vi "Construct.vi"(8 "error in (no error)":errorcluster, 11 "gRPCid":T1) -> (0 "error out":errorcluster, 3 "GRPCMessage out":refnum<class "GRPCMessage.lvclass">)   [LabVIEW 2019, in "MicronGRPCServer.lvlib" / "GRPCMessage.lvclass"]
uses:
  GRPCMessage.lvclass
  <vilib>/gRPC/LabVIEW gRPC Library/Shared/grpcId.ctl
  GRPCMessage.lvclass/GRPCMessage.ctl
  Service/Generated/MicronGRPCGeneratedServer/RPC Service/MicronGRPC/MicronGRPC.lvclass
  <vilib>/gRPC/LabVIEW gRPC Library/grpc-lvsupport-release.lvlib
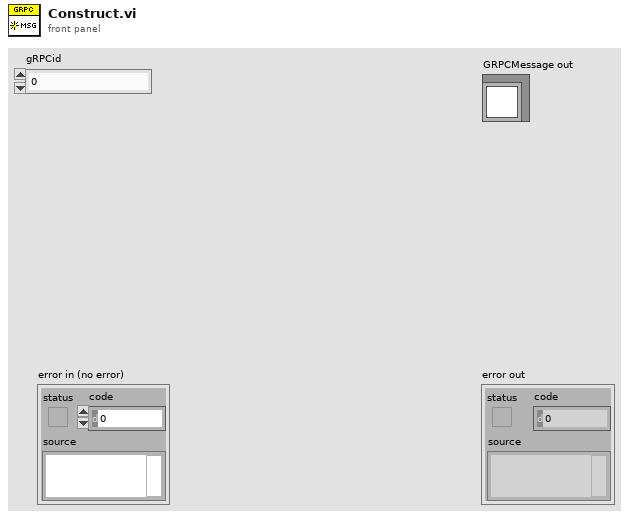
[diagram p1: front panel]
types:
  T1 = typedef "grpc-lvsupport-release.lvlib/grpcId.ctl" = u64
  T2 = typedef "MicronGRPCGeneratedServer.lvlib/micronGrpc_MessageRequest.ctl" = cluster{"command":string, "payload":string}
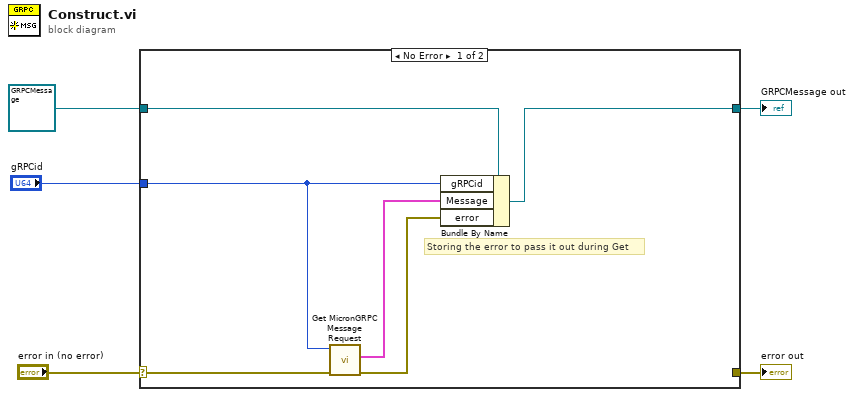
[diagram p0: block diagram]
diagram:
  n1 = case shown="No Error" "error in (no error)" {
    selector: "error in (no error)" -> [w8 w13]
    tunnel: [_ w13] -> w4
    tunnel: [w10 w12] -> w2
    tunnel: refnum<class "GRPCMessage.lvclass"> refnum ("GRPCMessage in") -> [w11 w12]
    tunnel: "gRPCid" -> [w9 _]
    frame No Error {
      # "Storing the error to pass it out during Get"
      n2 = call "Get MicronGRPC Message Request.vi"("error in (no error)"=w8, "gRPCid"=w9) -> ("error out"=w6:errorcluster, "Message Data"=w7:T2)  [unwired: 7 in, 1 out]
      n3 = Bundle By Name(cluster=w11, "gRPCid"=w9, "Message"=w7, "error"=w6) -> (w10:refnum<class "GRPCMessage.lvclass">)
    }
    frame Error {
    }
  }
  "error out" <- w4
  "GRPCMessage out" <- w2
